vi "Date Clicked.vi"(8 "Display State In":cluster{"Month":i32, "Day":i32, "Year":i32}, 10 "Coords":cluster{"Horizontal":i32, "Vertical":i32}, 11 "Dates":refnum<vi>) -> (0 "Display State Out":cluster{"Month":i32, "Day":i32, "Year":i32})   [LabVIEW 2019, in "Custom Calendar.xctl"]
uses:
  Custom Calendar.xctl
  <vilib>/Utility/miscctls.llb/LVRowAndColumnTypeDef.ctl
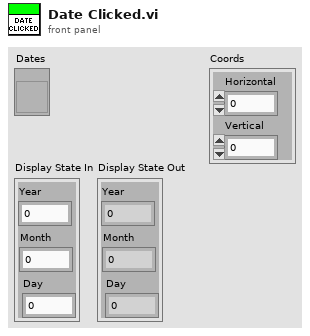
[diagram p1: front panel]
types:
  T1 = typedef "LVRowAndColumnTypeDef.ctl" = cluster{"Row":i32, "Column":i32}
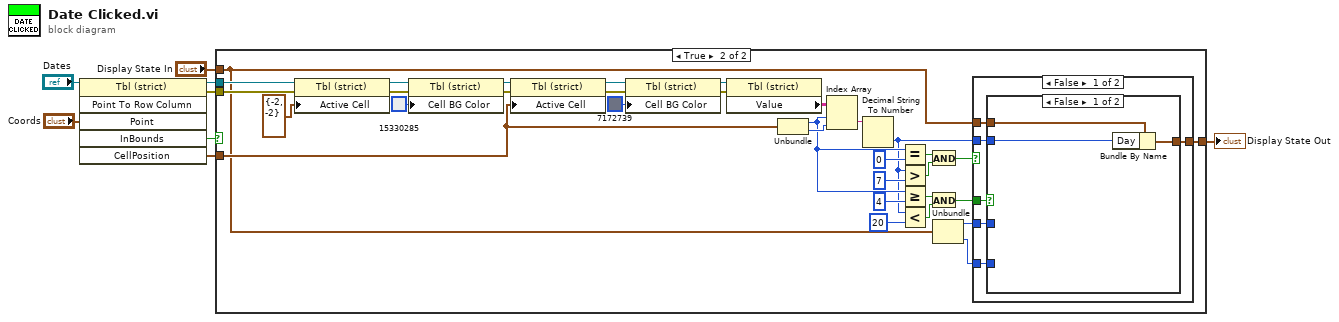
[diagram p0: block diagram]
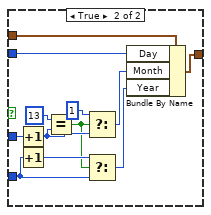
[diagram p3: hidden frame]
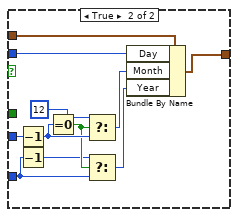
[diagram p4: hidden frame]
diagram:
  n1 = invoke class="Tbl (strict)" method="Point To Row Column"(reference="Dates", "Point"="Coords") -> (reference out=w2:refnum<vi>, error out=w1:errorcluster, "InBounds"=w4:bool, "CellPosition"=w5:T1)  [unwired: 4 in, 2 out]
  n2 = case shown="True" w4 {
    tunnel: "Display State In" -> [w9 w23]
    tunnel: w5 -> [_ w27]
    tunnel: [w9 w33] -> w3
    tunnel: w2 -> [_ w30]
    tunnel: w1 -> [_ w29]
    frame False {
    }
    frame True {
      n3 = property on="Property Node" class="Tbl (strict)"(reference=w30, error in=w29, "Active Cell"=T1 {"Row"=-2, "Column"=-2} ("Active Cell:Active Cell")) -> (reference out=w36:refnum<vi>, error out=w41:errorcluster)
      n4 = property on="Property Node" class="Tbl (strict)"(reference=w36, error in=w41, "Cell BG Color"=u32 15330285 ("Active Cell:Cell Background Color")) -> (reference out=w35:refnum<vi>, error out=w42:errorcluster)
      n5 = property on="Property Node" class="Tbl (strict)"(reference=w35, error in=w42, "Active Cell"=w27) -> (reference out=w34:refnum<vi>, error out=w37:errorcluster)
      n6 = property on="Property Node" class="Tbl (strict)"(reference=w34, error in=w37, "Cell BG Color"=u32 7172739 ("Active Cell:Cell Background Color")) -> (reference out=w32:refnum<vi>, error out=w31:errorcluster)
      n7 = property on="Property Node" class="Tbl (strict)"(reference=w32, error in=w31) -> ("Value"=w28:string[][])  [unwired: 2 out]
      n8 = Unbundle(w27) -> ("Row"=w24:i32, "Column"=w26:i32)
      n9 = Index Array(array=w28, index (row)=w24, index (col)=w26) -> (element=w25:string)
      n10 = Decimal String To Number(string=w25) -> (number=w19:i32)  [unwired: 2 in, 1 out]
      n11 = Equal?(x=w24, y=0) -> (x = y?=w18:bool)
      n12 = Greater?(x=w19, y=7) -> (0:w17:bool)
      n13 = Greater Or Equal?(x=w24, y=4) -> (x >= y?=w15:bool)
      n14 = Less?(x=w19, y=20) -> (x < y?=w14:bool)
      n15 = And(x=w18, y=w17) -> (x .and. y?=w16:bool)
      n16 = And(x=w15, y=w14) -> (x .and. y?=w13:bool)
      n17 = Unbundle(w23) -> ("Month"=w12:i32, "Year"=w11:i32)  [unwired: 1 out]
      n18 = case shown="False" w16 {
        tunnel: [w46 w74] -> w33
        tunnel: w23 -> [w47 w73]
        tunnel: w19 -> [w48 w72]
        tunnel: w13 -> [w45 _]
        tunnel: w12 -> [w43 w71]
        tunnel: w11 -> [w44 w66]
        frame False {
          n19 = case shown="False" w45 {
            tunnel: w48 -> [w51 w55]
            tunnel: w47 -> [w50 w53]
            tunnel: [w49 w54] -> w46
            tunnel: w44 -> [_ w61]
            tunnel: w43 -> [_ w60]
            frame False {
              n20 = Bundle By Name(cluster=w50, "Day"=w51) -> (w49:cluster{"Month":i32, "Day":i32, "Year":i32})
            }
            frame True {
              n21 = Increment(x=w60) -> (x+1=w59:i32)
              n22 = Increment(x=w61) -> (x+1=w63:i32)
              n23 = Equal?(x=13 ("t"), y=w59) -> (x = y?=w58:bool)
              n24 = Select(t=1, s=w58, f=w59) -> (s? t:f=w52:i32)
              n25 = Select(t=w63, s=w58, f=w61) -> (s? t:f=w62:i32)
              n26 = Bundle By Name(cluster=w53, "Day"=w55, "Month"=w52, "Year"=w62) -> (w54:cluster{"Month":i32, "Day":i32, "Year":i32})
            }
          }
        }
        frame True {
          n27 = Decrement(x=w71) -> (x-1=w70:i32)
          n28 = Decrement(x=w66) -> (x-1=w67:i32)
          n29 = Equal To 0?(x=w70) -> (x = 0?=w68:bool)
          n30 = Select(t=12, s=w68, f=w70) -> (s? t:f=w65:i32)
          n31 = Select(t=w67, s=w68, f=w66) -> (s? t:f=w64:i32)
          n32 = Bundle By Name(cluster=w73, "Day"=w72, "Month"=w65, "Year"=w64) -> (w74:cluster{"Month":i32, "Day":i32, "Year":i32})
        }
      }
    }
  }
  "Display State Out" <- w3
